vi "athena FPGA globals.vi"() -> ()   [LabVIEW 2009]
panel:
  in  "system stop":bool
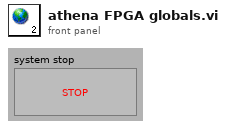
[diagram p1: front panel]
diagram:
